vi "week_one.vi"() -> ()   [LabVIEW 2017]
panel:
  out "Gauge":dbl(knob) scale=0.0..10.0
  in  "data":dbl
  out "data 2":dbl
  out "Gauge 2":dbl(knob) scale=0.0..10.0
  in  "stop":bool
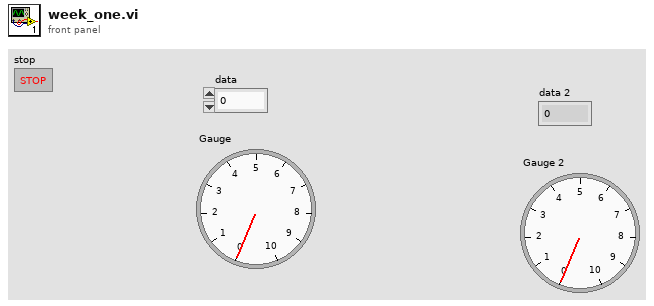
[diagram p1: front panel]
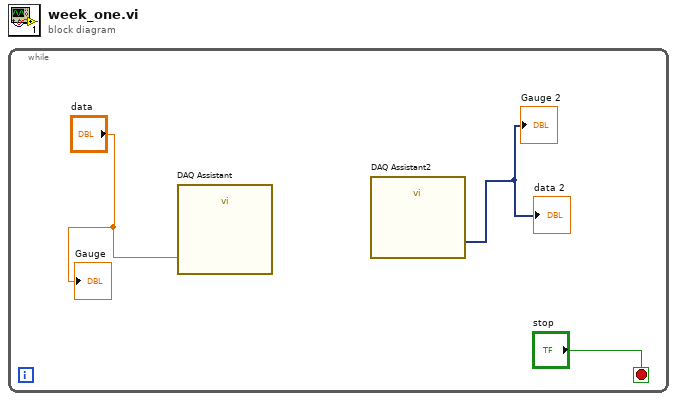
[diagram p0: block diagram]
diagram:
  n1 = while {
    stop <- "stop" stop-if-true
    n2 = call "DAQ Assistant"("data"="data") -> ()  [unwired: 17 in, 2 out]
    n3 = call "DAQ Assistant2"() -> ("data"=→"Gauge 2" →"data 2":dynamicdata)  [unwired: 17 in, 2 out]
    "Gauge" <- "data"
  }
